vi "计数器值转换成对应的物理值.vi"(8 "错误输入":errorcluster caption="错误输入（无错误）", 9 "ctCode":u32, 10 "chNo":i32, 11 "设备句柄入":i32) -> (0 "错误输出":errorcluster, 1 "ctValue":dbl, 3 "设备句柄":i32=1)   [LabVIEW 2016]
uses:
  dll/em9636.dll
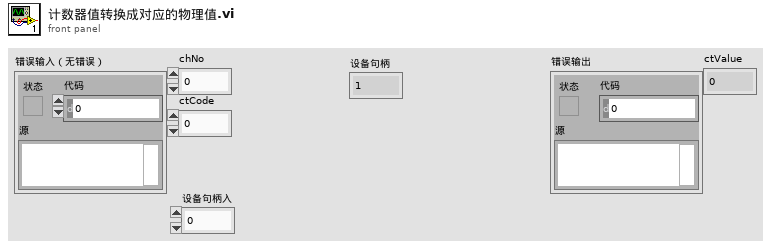
[diagram p1: front panel]
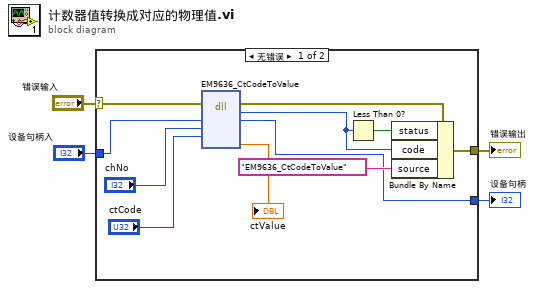
[diagram p0: block diagram]
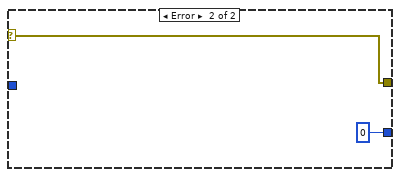
[diagram p2: hidden frame]
diagram:
  n1 = case shown="无错误" "错误输入" {
    selector: "错误输入" -> [w15 w17]
    tunnel: [w11 w17] -> w3
    tunnel: [w8 0 ("错误")] -> w2
    tunnel: "设备句柄入" -> [w9 _]
    frame No Error {
      n2 = dll-call lib="PTH2kabs CUsers\nAdministratorDesktopEM9636*EM9636系列_demo_labview(调用DLL方式)dll\nem9636.dll" fn="EM9636_CtCodeToValue"(error in=w15, "设备句柄"=w9, "chNo"="chNo", "ctCode"="ctCode") -> (error out=w13:errorcluster, "错误"=w10:i32, "设备句柄"=w8:i32, "ctValue"=→"ctValue":dbl)  [unwired: 5 in, 1 out]
      n3 = Less Than 0?(x=w10) -> (x < 0?=w12:bool)
      n4 = Bundle By Name(cluster=w13, "status"=w12, "code"=w10, "source"="EM9636_CtCodeToValue") -> (w11:errorcluster)
    }
    frame Error {
    }
  }
  "错误输出" <- w3
  "设备句柄" <- w2
